vi "Running.vi"(8 "error in (no error)":errorcluster caption="entrée d'erreur (pas d'erreur)", 11 "Process (Default) en entrée":refnum<class "Process (Default).lvclass">) -> (0 "error out":errorcluster caption="sortie d'erreur", 3 "Process (Default) en sortie":refnum<class "Process (Default).lvclass">)   [LabVIEW 2020, in "Library Instrument & Equipement.lvlib" / "Process (Default).lvclass"]
uses:
  Process (Default).lvclass
  Process (Default).lvclass/Process (Default).ctl
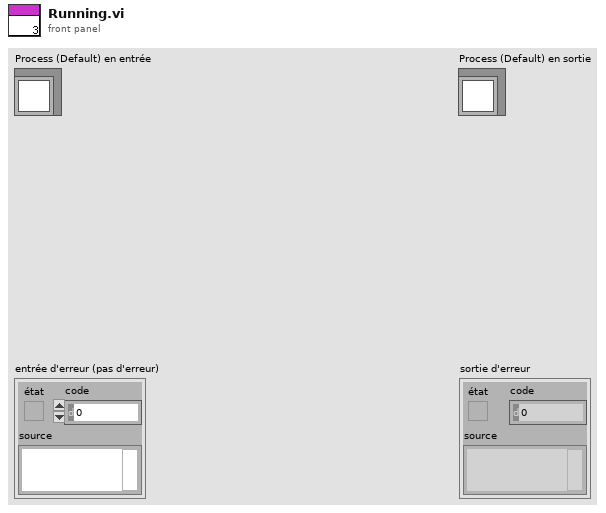
[diagram p1: front panel]
types:
  T1 = cluster{"Standard Output":string, "Process_is_Finish":bool}
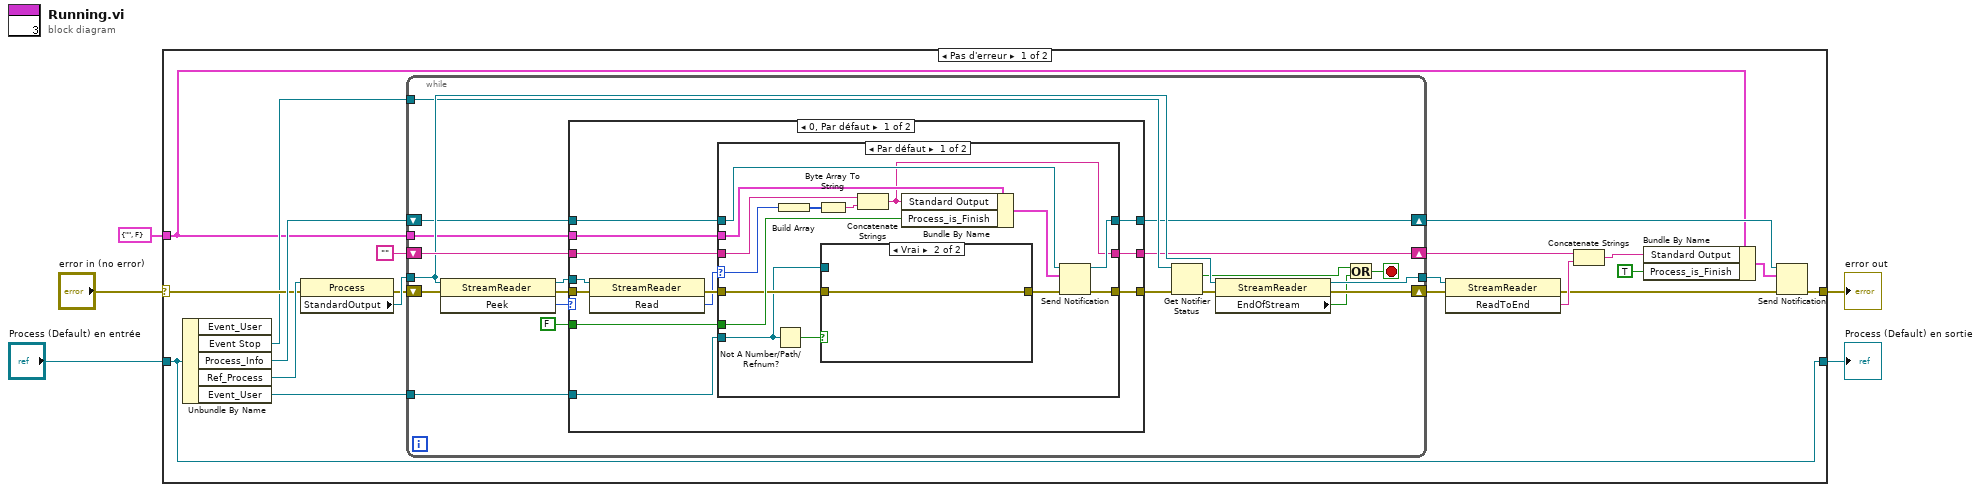
[diagram p0: block diagram]
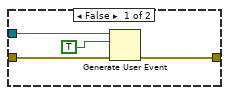
[diagram p2: hidden frame]
diagram:
  n1 = case shown="Pas d'erreur" "error in (no error)" {
    selector: "error in (no error)" -> [w13 w85]
    tunnel: [w15 w85] -> w4
    tunnel: [w22 w84] -> w2
    tunnel: "Process (Default) en entrée" -> [w22 w84]
    tunnel: T1 {"Standard Output"="", "Process_is_Finish"=FALSE} ("notification") -> [w7 _]
    frame No Error {
      n2 = Unbundle By Name(w22) -> ("Event Stop"=w8:refnum<notifier>, "Process_Info"=w16:refnum<notifier>, "Ref_Process"=w21:refnum<k24>, "Event_User"=w6:refnum<user-event>)  [unwired: 1 out]
      n3 = property class="Process"(reference=w21, error in=w13) -> (error out=w23:errorcluster, "StandardOutput"=w24:refnum<k24>)  [unwired: 1 out]
      n4 = while {
        tunnel: w24 -> [w41]
        shift-right: [w31] -> w17
        shift-left: "" -> [w42]
        shift-right: [w40] -> w19
        shift-left: w23 -> [w39]
        tunnel: [w38] -> w20
        shift-right: [w28] -> w14
        shift-left: w16 -> [w29]
        tunnel: w8 -> [w34]
        tunnel: w7 -> [w32]
        tunnel: w6 -> [w26]
        stop <- w36 stop-if-true
        n5 = invoke class="StreamReader" method="Peek"(reference=w41, error in=w39) -> (reference out=w45:refnum<k24>, error out=w44:errorcluster, "Peek"=w43:i32)  [unwired: 1 in]
        n6 = case shown="0, Par défaut" w43 {
          tunnel: [w47 w83] -> w31
          tunnel: w42 -> [w57 w83]
          tunnel: [w55 w82] -> w35
          tunnel: w45 -> [w53 _]
          tunnel: w44 -> [w52 w82]
          tunnel: w32 -> [w51 _]
          tunnel: FALSE ("Process_is_Finish") -> [w50 _]
          tunnel: w29 -> [w49 w81]
          tunnel: [w48 w81] -> w28
          tunnel: w26 -> [w46 _]
          frame 0, Default {
            n7 = invoke class="StreamReader" method="Read"(reference=w53, error in=w52) -> (error out=w56:errorcluster, "Read"=w54:i32)  [unwired: 1 in, 1 out]
            n8 = case shown="Par défaut" w54 {
              selector: w54 -> [w72 _]
              tunnel: w56 -> [w61 w79]
              tunnel: [w62 w79] -> w55
              tunnel: w57 -> [w69 w80]
              tunnel: [w63 w80] -> w47
              tunnel: w51 -> [w67 _]
              tunnel: w50 -> [w66 _]
              tunnel: w49 -> [w65 w78]
              tunnel: [w64 w78] -> w48
              tunnel: w46 -> [w59 _]
              frame Default {
                n9 = Not A Number/Path/Refnum?(number/path/refnum=w59) -> (NaN/Path/Refnum?=w58:bool)
                n10 = Build Array(w72) -> (w71:i32[])
                n11 = Byte Array To String(unsigned byte array=w71) -> (string=w70:string)
                n12 = case shown="Vrai" w58 {
                  tunnel: w61 -> [w76 w77]
                  tunnel: [w75 w77] -> w60
                  tunnel: w59 -> [w74 _]
                  frame False {
                    n13 = Generate User Event(user event=w74, event data cluster=TRUE ("données d'événement"), error in=w76) -> (error out=w75:errorcluster)  [unwired: 1 in, 1 out]
                  }
                  frame True {
                  }
                }
                n14 = Concatenate Strings(w69, w70) -> (w63:string)
                n15 = Bundle By Name(cluster=w67, "Standard Output"=w63, "Process_is_Finish"=w66) -> (w68:T1)
                n16 = Send Notification(notification=w68, notifier=w65, error in (no error)=w60) -> (notifier out=w64:refnum<notifier>, error out=w62:errorcluster)
              }
              frame -1 {
              }
            }
          }
          frame -1 {
          }
        }
        n17 = Get Notifier Status(notifier=w34, error in (no error)=w35) -> (current notification=w33:bool, error out=w27:errorcluster)  [unwired: 3 out]
        n18 = property class="StreamReader"(reference=w41, error in=w27) -> (reference out=w38:refnum<k24>, error out=w40:errorcluster, "EndOfStream"=w37:bool)
        n19 = Or(x=w33, y=w37) -> (x .or. y?=w36:bool)
      }
      n20 = invoke class="StreamReader" method="ReadToEnd"(reference=w20, error in=w19) -> (error out=w9:errorcluster, "ReadToEnd"=w18:string)  [unwired: 1 in, 1 out]
      n21 = Concatenate Strings(w17, w18) -> (w12:string)
      n22 = Bundle By Name(cluster=w7, "Standard Output"=w12, "Process_is_Finish"=TRUE) -> (w11:T1)
      n23 = Send Notification(notification=w11, notifier=w14, error in (no error)=w9) -> (error out=w15:errorcluster)  [unwired: 1 out]
    }
    frame Error {
    }
  }
  "error out" <- w4
  "Process (Default) en sortie" <- w2
